vi "Wind Farm #3 Cluster.vi"() -> (0 "Cluster":T2)   [LabVIEW 2011]
doc: "This is the cluster for Wind Farm #4.\n\nAAL 9/09"
uses:
  SEQ Solution/Controls/Wind Turbine DataRef.ctl
  SEQ Solution/Controls/Wind Turbine Data.ctl
  SEQ Solution/SEQ - Solution.lvlib
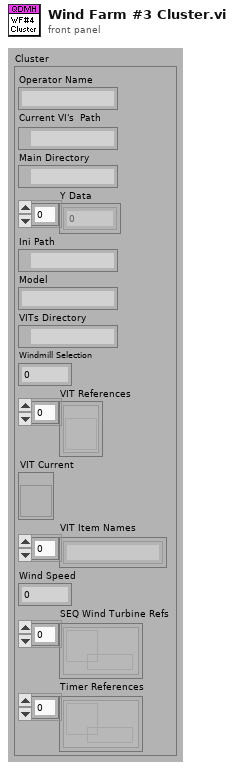
[diagram p1: front panel]
types:
  T1 = typedef "SEQ - Solution.lvlib/Wind Turbine DataRef.ctl" = refnum<queue>
  T2 = cluster{"Operator Name":string, "Current VI's  Path":path, "Main Directory":path, "Y Data":dbl[], "Ini Path":path, "Model":string, "VITs Directory":path, "Windmill Selection":i32, "VIT References":refnum<vi>[], "VIT Current":refnum<vi>, "VIT Item Names":string[], "Wind Speed":dbl, "SEQ Wind Turbine Refs":T1[], "Timer References":refnum<data-value>[]}
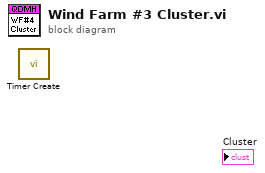
[diagram p0: block diagram]
diagram:
  n1 = call "Timer Create.vi"() -> ()  [unwired: 10 in, 2 out]
